vi "Set Manifestation Ancestor Path.vi"(10 "Manifestation Ancestor Path":path, 11 "Manifestation Writer in":refnum<class "Manifestation Writer.lvclass">) -> (3 "Manifestation Writer out":refnum<class "Manifestation Writer.lvclass">)   [LabVIEW 2013, in "Manifestation Writer.lvclass"]
uses:
  Manifestation Writer.lvclass
  Manifestation Writer.lvclass/Manifestation Writer.ctl
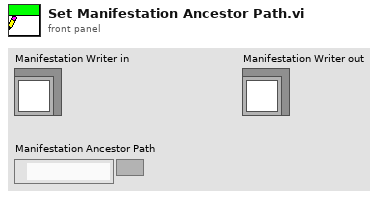
[diagram p1: front panel]
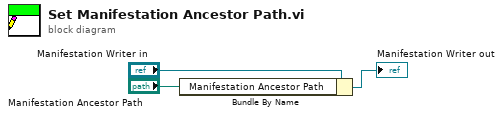
[diagram p0: block diagram]
diagram:
  n1 = Bundle By Name(cluster="Manifestation Writer in", "Manifestation Ancestor Path"="Manifestation Ancestor Path") -> (→"Manifestation Writer out":refnum<class "Manifestation Writer.lvclass">)
